vi "Get RefreshTime Notifier.vi"(8 "error in (no error)":errorcluster, 11 "Transport in":refnum<class "Transport.lvclass">) -> (0 "error out":errorcluster, 1 "valid?":bool, 2 "refresh (ms)":u32, 3 "Transport out":refnum<class "Transport.lvclass">)   [LabVIEW 2019, in "Transport.lvclass"]
uses:
  Transport.lvclass
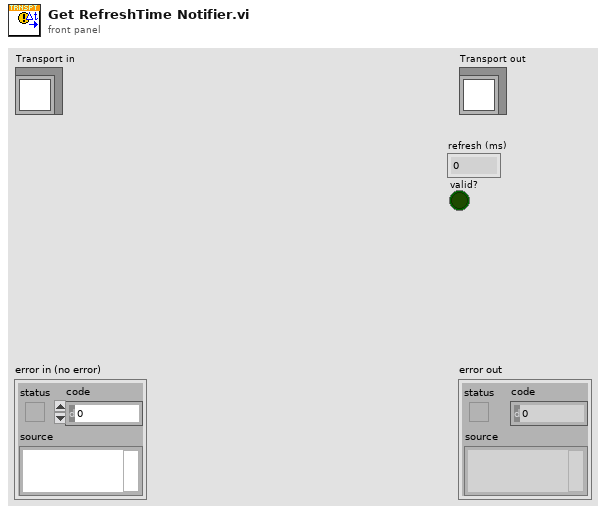
[diagram p1: front panel]
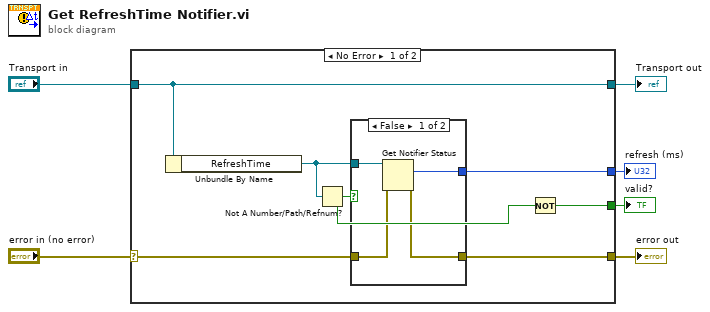
[diagram p0: block diagram]
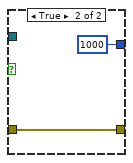
[diagram p2: hidden frame]
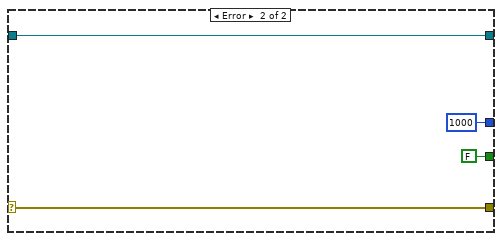
[diagram p3: hidden frame]
diagram:
  n1 = case shown="No Error" "error in (no error)" {
    selector: "error in (no error)" -> [w13 w22]
    tunnel: [w12 w22] -> w5
    tunnel: [w10 w23] -> w3
    tunnel: "Transport in" -> [w10 w23]
    tunnel: [w11 u32 1000 ("refresh (ms)")] -> w2
    tunnel: [w7 FALSE] -> w1
    frame No Error {
      n2 = Unbundle By Name(w10) -> ("RefreshTime"=w9:refnum<notifier>)
      n3 = Not A Number/Path/Refnum?(number/path/refnum=w9) -> (NaN/Path/Refnum?=w8:bool)
      n4 = case shown="False" w8 {
        tunnel: w13 -> [w17 w19]
        tunnel: [w16 w19] -> w12
        tunnel: [w15 u32 1000 ("refresh (ms)")] -> w11
        tunnel: w9 -> [w14 _]
        frame False {
          n5 = Get Notifier Status(notifier=w14, error in (no error)=w17) -> (current notification=w15:u32, error out=w16:errorcluster)  [unwired: 3 out]
        }
        frame True {
        }
      }
      n6 = Not(x=w8) -> (.not. x?=w7:bool)
    }
    frame Error {
    }
  }
  "error out" <- w5
  "Transport out" <- w3
  "refresh (ms)" <- w2
  "valid?" <- w1
